vi "daqio_Create_Device.vi"(8 "error in":errorcluster, 9 "Device Label":string, 10 "Device Key":string, 11 "daq.io type in":T1={"daq.io ref"=refnum, "daq.io API Base"="http://dashboard.daq.io/api/v1", "Device Key"="", "Account ID"="", "online"=TRUE, "SSL"=TRUE}) -> (0 "error out":errorcluster, 3 "daq.io type out":T1={"daq.io ref"=refnum, "daq.io API Base"="http://dashboard.daq.io/api/v1", "Device Key"="", "Account ID"="", "online"=TRUE, "SSL"=TRUE})   [LabVIEW 2013, in "daqio minimal.lvlib"]
doc: "This VI creates a new device for a given Device Key."
uses:
  daqio minimal.lvlib
  <vilib>/Easy HTTP Client/HTTP Header.ctl
  _typedefs/daqio-Type.ctl
  <vilib>/httpClient/ClientHandle.ctl
  _typedefs/daqio-Device-minimum.ctl
  <vilib>/Easy HTTP Client/Easy HTTP.lvlib
  <vilib>/httpClient/LabVIEWHTTPClient.lvlib
panel:
  out "JSON string":string
  out "headers":T3[](array[typedef])
  out "body":string
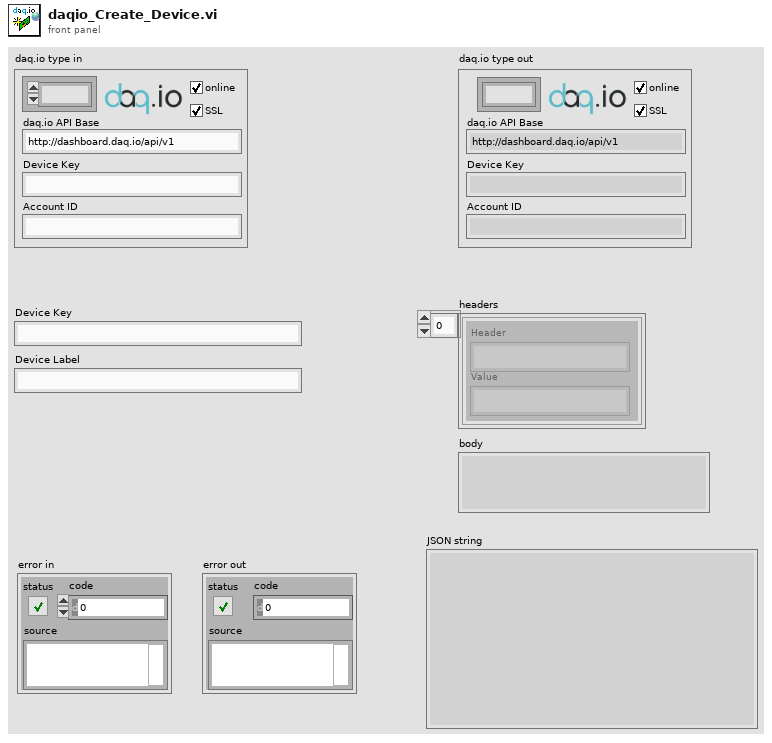
[diagram p1: front panel]
types:
  T1 = typedef "daqio minimal.lvlib/daqio-Type.ctl" = cluster{"daq.io ref":T2, "daq.io API Base":string, "Device Key":string, "Account ID":string, "online":bool, "SSL":bool}
  T2 = typedef "LabVIEWHTTPClient.lvlib/ClientHandle.ctl" = refnum<k1>
  T3 = typedef "Easy HTTP.lvlib/HTTP Header.ctl" = cluster{"Header":string, "Value":string}
  T4 = typedef "daqio minimal.lvlib/daqio-Device-minimum.ctl" = cluster{"label":string, "key":string, "tags":cluster{"key":string, "value":string}[]}
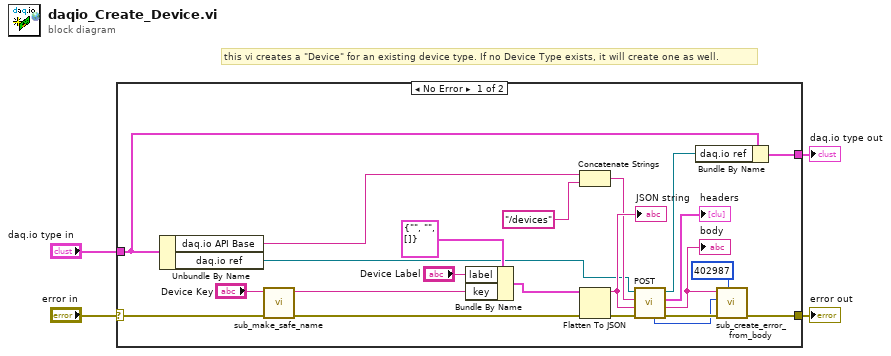
[diagram p0: block diagram]
diagram:
  # "this vi creates a \"Device\" for an existing device type. If no Device Type exists, it will create one as well."
  n1 = case shown="No Error" "error in" {
    selector: "error in" -> [w13 w26]
    tunnel: "daq.io type in" -> [w12 w27]
    tunnel: [w16 w27] -> w3
    tunnel: [w11 w26] -> w2
    frame No Error {
      n2 = Unbundle By Name(w12) -> ("daq.io API Base"=w6:string, "daq.io ref"=w5:T2)
      n3 = call "sub_make_safe_name.vi"("Input String"="Device Key") -> ("Safe Output String"=w14:string)  [unwired: 10 in]
      n4 = Bundle By Name(cluster=T4 {"label"="", "key"="", "tags"=[]}, "label"="Device Label", "key"=w14) -> (w17:T4)
      n5 = Concatenate Strings(w6, "/devices" ("string")) -> (w18:string)
      n6 = Flatten To JSON(anything=w17, error in (no error)=w13) -> (JSON string=w23:string, 11:w25:errorcluster)  [unwired: 1 in]
      "JSON string" <- w23
      n7 = call <vilib>:"POST.vi"("error in (no error)"=w25, "data"=w23, "url"=w18, "client handle"=w5) -> ("error out"=w10:errorcluster, "body"=w8:string, "headers"=→"headers":T3[], "client handle out"=w21:T2, "HTTP Response Code"=w9:i32)  [unwired: 3 in]
      "body" <- w8
      n8 = Bundle By Name(cluster=w12, "daq.io ref"=w21) -> (w16:T1)
      n9 = call "sub_create_error_from_body.vi"("error code"=402987, "error in (no error)"=w10, "http code"=w9, "body"=w8) -> ("error out"=w11:errorcluster)  [unwired: 7 in]
    }
    frame Error {
    }
  }
  "error out" <- w2
  "daq.io type out" <- w3
